vi "AlliGator Get Optimal IRF from Decay v2.vi"(8 "error in (no error)":errorcluster, 11 "Selected Plot Info":T4={"Multiplot XY Graph"=refnum, "Mouse Coordinates"={"Horizontal"=0, "Vertical"=0}, "Plot Index"=-1}) -> (0 "Error Out":errorcluster, 1 "Message Style":T2={"Font"="Consolas", "Text Color"=enum."Black", "Text Background Color"=enum."White", "Text Style"=enum."Regular", "Font Size (Points)"=10.0, "Text Alignment"=0} {"Text Alignment" items=["Left", "Right", "Center"]}, 2 "Message":string, 3 "Extracted IRF":cluster{"t Array":dbl[], "IRF Array":dbl[]})   [LabVIEW 2021, in "AlliGator Decay Analysis.lvlib" / "AlliGator IRF.lvlib"]
doc: "Extract IRF from single-exponential decay by deconvolution and optimization of the time constant."
uses:
  AlliGator IRF.lvlib
  Graphs/XY Graph/XY Graph Selected Plot Info.ctl
  Graphs/XY Graph/XY Graph Refnum.ctl
  <vilib>/Utility/miscctls.llb/LVPoint32TypeDef.ctl
  Rich Text Box/Text Formatting.ctl
  Rich Text Box/Text Colors.ctl
  AlliGator Settings List.ctl
  AlliGator IRF Optimization Controls.ctl
  AlliGator IRF Deconvolution Metrics.ctl
  Fits/IRF(X)PSED/IRF(X)PSED Fixed Parameters v3.ctl
  Fits/IRF(X)PSED/IRF(X)PSED Extraction Options.ctl
  Fits/IRF(X)PSED/Fourier Series Smoothing Option.ctl
  Fits/IRF(X)PSED/Fourier Series Truncation.ctl
  Fits/IRF(X)PSED/IRF Extraction Method.ctl
  Variant/Variant to Data/Variant to I32.vi
  Graphs/XY Graph/XY Graph Add Single Plot with Name.vi
  Graphs/XY Graph/XY Graph Add-Ons.lvlib
  AlliGator Settings.lvlib
  Notebook/Notebook.lvlib
  Fits/Fits.lvlib
  Variant/Variant to Data/Variant to Data.lvlib
  Rich Text Box/Rich Text Box.lvlib
panel:
  in  "Tab Control":T1(tab)
  out "Optimization Graph":cluster{"X Array":dbl[], "Y Array":dbl[]}[](graph)
  out "Power Spectrum Graph":dbl[][](graph)
  in  "Plot Names":string[](array[string])=["Tail Average", "Tail Average SG", "Tail SDV", "Tail SDV S-G", "Tail Max", "Tail Max S-G", "Tail SDV x Average", "Tail SDV x Average S-G", "Slope"]
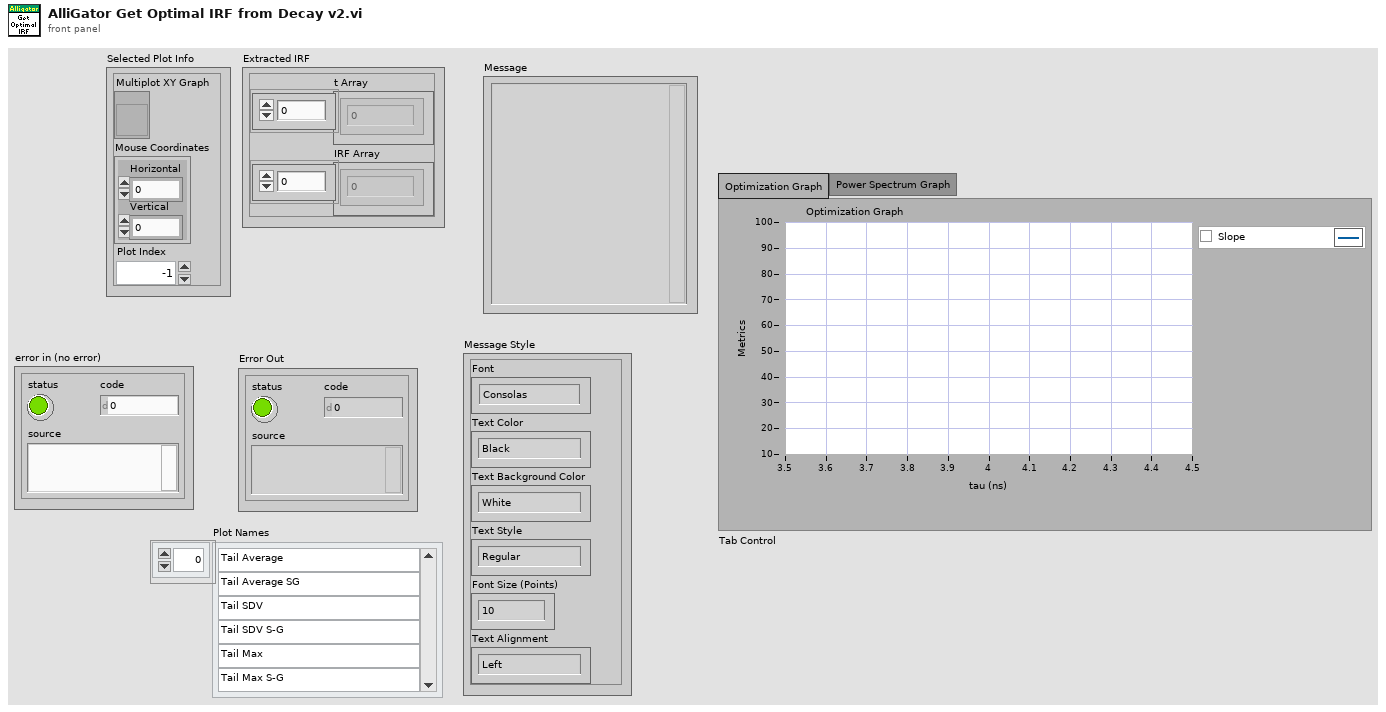
[diagram p1: front panel]
types:
  T1 = enum32{"Optimization Graph", "Power Spectrum Graph"}
  T2 = typedef "Rich Text Box.lvlib/Text Formatting.ctl" = cluster{"Font":string, "Text Color":T3, "Text Background Color":T3, "Text Style":enum16{"Regular", "Bold", "Italic", "Underline", "Strikeout"}, "Font Size (Points)":dbl, "Text Alignment":i32}
  T3 = typedef "Rich Text Box.lvlib/Text Colors.ctl" = enum16{"Unchanged", "Black", "Blue", "Brown", "Gray", "Green", "Orange", "Pink", "Red", "White"}
  T4 = typedef "XY Graph Add-Ons.lvlib/XY Graph Selected Plot Info.ctl" = cluster{"Multiplot XY Graph":T5, "Mouse Coordinates":T6, "Plot Index":i32}
  T5 = typedef "XY Graph Add-Ons.lvlib/XY Graph Refnum.ctl" = refnum<vi>
  T6 = typedef "LVPoint32TypeDef.ctl" = cluster{"Horizontal":i32, "Vertical":i32}
  T7 = typedef "Fits.lvlib/IRF(X)PSED Extraction Options.ctl" = cluster{"Time Constant for IRF Extraction":dbl[unit], "IRF Order":i32, "Fourier Series Smoothing":T8, "Noise Threshold":dbl, "Smoothing Width":dbl, "Fourier Series Truncation":T9, "Truncation Order":i32, "Save Power Spectrum":bool, "Smoothing":bool, "Smoothing Parameter":dbl, "Smoothing Order":u32, "Method":T10}
  T8 = typedef "Fits.lvlib/Fourier Series Smoothing Option.ctl" = enum16{"None", "Lanczos Factors", "Fejer Summation"}
  T9 = typedef "Fits.lvlib/Fourier Series Truncation.ctl" = enum16{"Automatic", "Fixed"}
  T10 = typedef "Fits.lvlib/IRF Extraction Method.ctl" = enum16{"Direct", "Topless", "Toeplitz"}
  T11 = typedef "Fits.lvlib/IRF(X)PSED Fixed Parameters v3.ctl" = cluster{"order":i32, "T":dbl, "Time Constant Array":dbl[], "{S_k, C_k, phi_k, e_k} arrays":cluster{"S_k Array":dbl[], "C_k Array":dbl[], "phi_k Array":dbl[], "e_k Array":dbl[]}, "IRF Extraction Options":T7}
  T12 = typedef "AlliGator Settings.lvlib/AlliGator Settings List.ctl" = enum16{"GUI:Visible Settings Tab", "GUI:Last Run Version", "Source Image:Use Image Histogram for Contrast", "Source Image:Low Count Pixels Rejection Options", "Source Image:High Count Pixels Rejection Options", "Source Image:Use Image Brightness", "Source Image:Blend Overlay with Image Background", "Source Image:Use Fixed ROI Diameter", "Source Image:ROI Diameter", "Source Image:ROI Center Color", "Source Image:Peak Threshold", "Source Image:Intensity Threshold", "Source Image:Image Binning Options", "Source Image:Image Smoothing Options", "Source Image:Image Histogram Active", "Source Image:Invert Binary Mask", "Source Image:Hot Pixel Removal", "Source Image:Overlay Analyzed ROI Center", "Source Image:Auto-Adjust Contrast", "Source Image:Histogram Lower Percentile", "Source Image:Histogram Upper Percentile", "Source Image:Save Source Image", "Source Image:Scale Bar Options", "Source Image:Image Resolution (Pixel Size)", "Source Image:Flatfield Correction", "Data Information:Gate Width", "Data Information:Nanotime Gate Separation", "Data Information:Macrotime Gate Separation", "Data Information:Gate Step", "Data Information:# Gates", "Data Information:Gate Image Exposure", "Data Information:Gate Image Integration", "Data Information:Gates to Skip", "Data Information:Gates to Keep", "Data Information:Define Gates to", "Data Information:Channel Name", "Data Information:Available Channel Names", "Data Information:Channel Arithmetic", "Data Information:Background File Subtraction", "Data Information:Background File", "Data Information:Background Scaling Factor", "Data Information:Background Pile-up Correction", "Data Information:Background Pixel Well Capacity", "Data Information:Laser Period", "Data Information:SYNC Period", "Data Information:Pile-up Correction", "Data Information:Pixel Well Capacity", "Data Information:Dataset Scaling Factor", "Fluorescence Decay_Decay Pre-Processing:Reverse Gates", "Fluorescence Decay_Decay Pre-Processing:Verbose Decay Pre-Processing", "Fluorescence Decay_Decay Pre-Processing:Use Decay Pre-Processing", "Fluorescence Decay_Decay Pre-Processing:Background Subtraction", "Fluorescence Decay_Decay Pre-Processing:Background Definition Range", "Fluorescence Decay_Decay Pre-Processing:Baseline Subtraction Method", "Fluorescence Decay_Decay Pre-Processing:Operations Order", "Fluorescence Decay_Decay Pre-Processing:Smoothing Parameter", "Fluorescence Decay_Decay Pre-Processing:Shift Decay", "Fluorescence Decay_Decay Pre-Processing:Decay Shift Parameters", "Fluorescence Decay_Decay Pre-Processing:Fold Decay", "Fluorescence Decay_Decay Pre-Processing:# Folds", "Fluorescence Decay_Decay Pre-Processing:1-Normalize Decay", "Fluorescence Decay_Decay Pre-Processing:[0-1]-Normalize Decay", "Fluorescence Decay_Decay Pre-Processing:Smoothen Decay", "Fluorescence Decay_Decay Pre-Processing:Extrapolate Decay", "Fluorescence Decay_Decay Pre-Processing:Use Periodicity", "Fluorescence Decay_Decay Pre-Processing:Use Cursors", "Fluorescence Decay_Decay Pre-Processing:Tail Fraction", "Fluorescence Decay_Decay Pre-Processing:Head Fraction", "Fluorescence Decay_Decay Pre-Processing:Additional Points", "Fluorescence Decay_Decay Pre-Processing:Straighten Decay", "Fluorescence Decay_Decay Pre-Processing:Constant Background", "Fluorescence Decay_Decay Pre-Processing:Pixel-Normalize Decay", "Fluorescence Decay_Advanced Analysis:Extract IRF instead of Decay", "Fluorescence Decay_Advanced Analysis:IRF Extraction Options", "Fluorescence Decay_Advanced Analysis:IRF Optimization Options", "Fluorescence Decay_Advanced Analysis:Square Pulse Options", "Fluorescence Decay_Advanced Analysis:IRF Order", "Fluorescence Decay_Advanced Analysis:IRF Time Constants", "Fluorescence Decay_Advanced Analysis:Wavelet Analysis Options", "Fluorescence Decay_Advanced Analysis:Average Lifetime Options", "Fluorescence Decay_Fit Options:Fit Options", "Fluorescence Decay_Fit Options:Use Legacy Fitting Approach", "Fluorescence Decay_Fit Options:Use Data Information Laser Period", "Fluorescence Decay_Fit Parameters:Displayed Fit Parameters", "Fluorescence Decay_Fit Parameters:Fit Parameter Constraints", "Fluorescence Decay_Fit Parameters:Export Tabulated Results", "Fluorescence Decay_Fit Parameters:MLE Baseline Offset Type", "Fluorescence Decay_Fit Parameters:MLE Baseline Offset", "Fluorescence Decay_Fit Parameters:Guess Parameter Names", "Fluorescence Decay_Fit Parameters:Guess Parameter Values", "Fluorescence Decay_Fit Parameters:Guess Parameters Options", "Fluorescence Decay_Styles:Show Last Decay Only", "Fluorescence Decay_Styles:Decay Graph Color Array", "Fluorescence Decay:Decay Graph Active", "Fluorescence Decay Statistics:Min Peak Value", "Fluorescence Decay Statistics:Reject Low Decay Peak Pixels", "Fluorescence Decay Statistics:Reject High Decay Peak Pixels", "Fluorescence Decay Statistics:Max Peak Value", "Time Traces:Use File Timestamp", "Time Traces:Time Step", "Time Traces:Use Intensity Correction File", "Time Traces:Intensity Correction File", "Phasor Plot:Phasor Plot Smoothing Options", "Phasor Plot:Phasor Plot Size", "Phasor Plot:Phasor Plot Graphics Options", "Phasor Plot:Cumulative Phasor Plot", "Phasor Plot:Use Phasor Brightness", "Phasor Plot:Blend Overlay with Phasor Background", "Phasor Plot:Save Phasor Plot", "Phasor Plot:Show References", "Phasor Plot:Phasor Ratio Decay Range", "Phasor Plot:Exponential Fading", "Phasor Plot:Phasor Ratio Reference Colors", "Phasor Plot:Reference Radius", "Phasor Plot:Show Color Map Vertices", "Phasor Plot:Phasor Plot Active", "Phasor Plot:Phasor Ratio Color Map Type", "Phasor Plot:Phasor Ratio Color Map", "Phasor Plot:Phasor Ratio Display Range", "Phasor Plot:Selected Image ROI(s)", "Phasor Plot:All Image ROIs", "Phasor Plot:Selected Phasor Plot ROI(s)", "Phasor Plot:All Phasor Plot ROIs", "Phasor Plot:Phasor Ratio Color-Coded Quantity", "Phasor Plot:Store Phasor Harmonics", "Phasor Plot:Draw Reference Segment", "Phasor Plot:User-Defined Quantity", "Phasor Graph:Phasor Frequency", "Phasor Graph:Phasor Ratio Type", "Phasor Graph:Pixel-level Phasor Computation", "Phasor Graph:Save Phasor Graph", "Phasor Graph:Phasor Graph Active", "Phasor Graph:Phasor SDV Options", "Phasor Calibration:Use Backup Calibration if needed", "Phasor Graph:Define Shortest Lifetime as", "Phasor Calibration:Backup Calibration Type", "Phasor Calibration:Calibration Type", "Phasor Calibration:Calibration Lifetime", "Phasor Calibration:Calibration Map Algorithm", "Single-Exponential Phasor Locus (SEPL):Gate Parameters", "Single-Exponential Phasor Locus (SEPL):User-defined Gate", "Single-Exponential Phasor Locus (SEPL):User-defined IRF", "Single-Exponential Phasor Locus (SEPL):Phasor Parameters", "Single-Exponential Phasor Locus (SEPL):Decay & IRF Parameters", "Single-Exponential Phasor Locus (SEPL):Display Parameters", "Lifetime Analysis:Decay Analysis Parameters", "Lifetime Analysis:Lifetime Map Active", "Plugins:Python Settings", "Miscellaneous:Verbose Mode", "Miscellaneous:Beep after Script", "Miscellaneous:Saved Image File Format", "Miscellaneous:Exported Gate Image Settings", "Miscellaneous:Include Loading in Timing", "Miscellaneous:Verbose Settings Mode", "Miscellaneous:Histogram Options", "Miscellaneous:Beep on Error", "Miscellaneous:# Logical Processors Used", "Miscellaneous:ROI Description Max Characters", "Miscellaneous:Verbose Error Mode", "Miscellaneous:Transparent Mask Color"}
  T13 = typedef "AlliGator Decay Analysis.lvlib/AlliGator IRF.lvlib/AlliGator IRF Optimization Controls.ctl" = cluster{"Search Range":dbl[unit], "Search Step":dbl[unit], "Tail threshold (%)":dbl, "Regularized IRF":bool, "Export Plot":bool, "Export Data":bool, "Smooth Metrics":bool, "S-G Side Points":i32, "S-G Polynomial Order":i32, "Metrics":T14}
  T14 = typedef "AlliGator Decay Analysis.lvlib/AlliGator IRF.lvlib/AlliGator IRF Deconvolution Metrics.ctl" = enum16{"Average", "SDV", "Max", "Average * SDV", "Slope"}
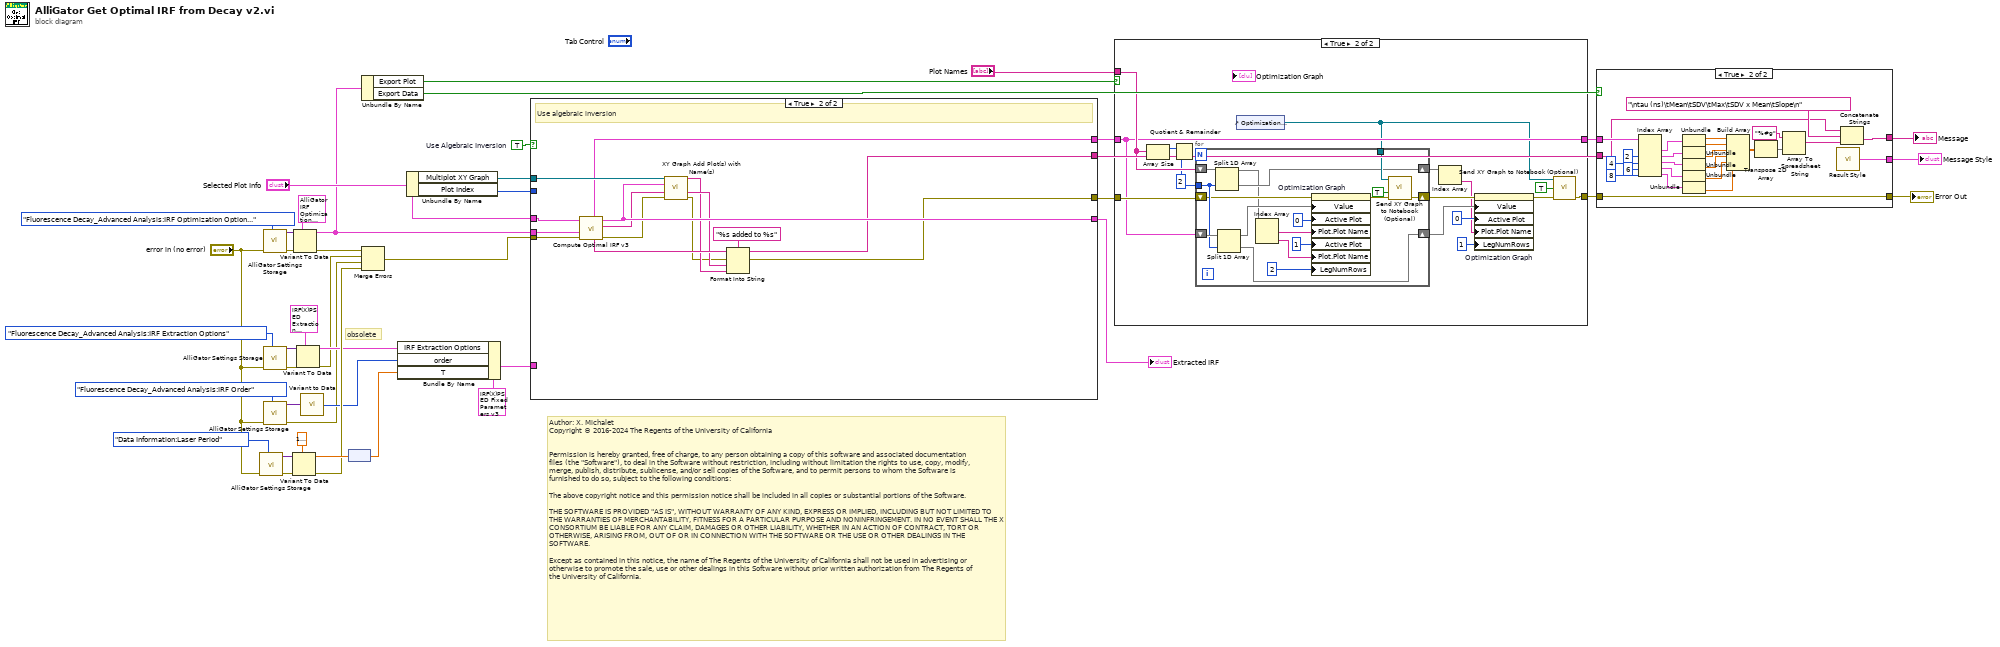
[diagram p0: block diagram]
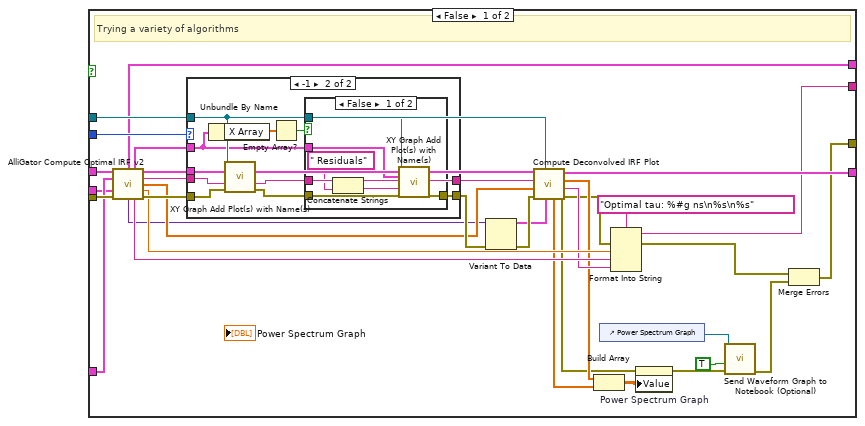
[diagram p4: hidden frame]
diagram:
  w13 = TRUE  # Use Algebraic Inversion
  # "Author: X. Michalet\nCopyright © 2016-2024 The Regents of the University of California\n \n\nPermission is hereby granted, free of charge, to any person obtaining a copy of this software and associated documentation files (the \"Software\"), to deal in the Software without restriction, including without limitation the rights to use, copy, modify, merge, publish, distribute, sublicense, and/or sell copies of the Software, and to permit persons to whom the Software is furnished to do so, subject to the following conditions:\n\nThe above copyright notice and this permission notice shall be included in all copies or substantial portions of the Software.\n\nTHE SOFTWARE IS PROVIDED \"AS IS\", WITHOUT WARRANTY OF ANY KIND, EXPRESS OR IMPLIED, INCLUDING BUT NOT LIMITED TO THE WARRANTIES OF MERCHANTABILITY, FITNESS FOR A PARTICULAR PURPOSE AND NONINFRINGEMENT. IN NO EVENT SHALL THE X CONSORTIUM BE LIABLE FOR ANY CLAIM, DAMAGES OR OTHER LIABILITY, WHETHER IN AN ACTION OF CONTRACT, TORT OR OTHERWISE, ARISING FROM, OUT OF OR IN CONNECTION WITH THE SOFTWARE OR THE USE OR OTHER DEALINGS IN THE SOFTWARE.\n\nExcept as contained in this notice, the name of The Regents of the University of California shall not be used in advertising or otherwise to promote the sale, use or other dealings in this Software without prior written authorization from The Regents of the University of California."
  # "obsolete"
  n1 = call "AlliGator Settings Storage.vi"("AlliGator Settings List"=AlliGator_Settings_List."Data Information:Laser Period", "Error In"="error in (no error)") -> ("Error Out"=w33:errorcluster, "Variant Data out"=w35:variant)  [unwired: 8 in]
  n2 = call "AlliGator Settings Storage.vi"("AlliGator Settings List"=AlliGator_Settings_List."Fluorescence Decay_Advanced Analysis:IRF Optimization Options", "Error In"="error in (no error)") -> ("Error Out"=w41:errorcluster, "Variant Data out"=w42:variant)  [unwired: 8 in]
  n3 = call "AlliGator Settings Storage.vi"("AlliGator Settings List"=AlliGator_Settings_List."Fluorescence Decay_Advanced Analysis:IRF Extraction Options", "Error In"="error in (no error)") -> ("Error Out"=w27:errorcluster, "Variant Data out"=w28:variant)  [unwired: 8 in]
  n4 = call "AlliGator Settings Storage.vi"("AlliGator Settings List"=AlliGator_Settings_List."Fluorescence Decay_Advanced Analysis:IRF Order", "Error In"="error in (no error)") -> ("Error Out"=w20:errorcluster, "Variant Data out"=w26:variant)  [unwired: 8 in]
  n5 = Variant To Data(error in=w33, type=dbl[unit] 1e-09 ("Time Constant"), Variant=w35) -> (data=w32:dbl[unit], error out=w30:errorcluster)
  n6 = Variant To Data(error in=w41, type=T13 {"Search Range"=1e-09, "Search Step"=1e-09, "Tail threshold (%)"=1.0, "Regularized IRF"=FALSE, "Export Plot"=FALSE, "Export Data"=FALSE, "Smooth Metrics"=FALSE, "S-G Side Points"=1, "S-G Polynomial Order"=3, "Metrics"=enum."Average"} ("IRF Optimization Control"), Variant=w42) -> (data=w12:T13, error out=w38:errorcluster)
  n7 = Variant To Data(error in=w27, type=T7 {"Time Constant for IRF Extraction"=4.08e-09, "IRF Order"=132, "Fourier Series Smoothing"=enum."Fejer Summation", "Noise Threshold"=0.1, "Smoothing Width"=0.1, "Fourier Series Truncation"=enum."Automatic", "Truncation Order"=0, "Save Power Spectrum"=FALSE, "Smoothing"=FALSE, "Smoothing Parameter"=0.0, "Smoothing Order"=1, "Method"=enum."Direct"} ("IRF Extraction Options"), Variant=w28) -> (data=w23:T7, error out=w21:errorcluster)
  n8 = call-poly "Variant to Data.vi"("Variant"=w26) -> ("Value"=w22:i32)  [unwired: 8 in]
  n9 = node(w32) -> (w19:dbl)
  n10 = Unbundle By Name(w12) -> ("Export Plot"=w9:bool, "Export Data"=w8:bool)
  n11 = Merge Errors(w38, w21, w20, w30) -> (w31:errorcluster)
  n12 = Bundle By Name(cluster=T11 {"order"=0, "T"=0.0, "Time Constant Array"=[], "{S_k, C_k, phi_k, e_k} arrays"={"S_k Array"=[], "C_k Array"=[], "phi_k Array"=[], "e_k Array"=[]}, "IRF Extraction Options"={"Time Constant for IRF Extraction"=1e-18, "IRF Order"=0, "Fourier Series Smoothing"=enum."None", "Noise Threshold"=0.0, "Smoothing Width"=0.0, "Fourier Series Truncation"=enum."Automatic", "Truncation Order"=0, "Save Power Spectrum"=FALSE, "Smoothing"=FALSE, "Smoothing Parameter"=0.0, "Smoothing Order"=1, "Method"=enum."Direct"}} ("IRF*PSED Fixed Parameters"), "IRF Extraction Options"=w23, "order"=w22, "T"=w19) -> (w15:T11)
  n13 = Unbundle By Name("Selected Plot Info") -> ("Multiplot XY Graph"=w16:T5, "Plot Index"=w17:i32)
  n14 = case shown="True" w13 {
    tunnel: "Selected Plot Info" -> [w75 w110]
    tunnel: [w74 w108] -> w37
    tunnel: w31 -> [w73 w111]
    tunnel: w17 -> [w72 _]
    tunnel: w16 -> [w71 w109]
    tunnel: [w66 w100] -> w10
    tunnel: w15 -> [w62 _]
    tunnel: w12 -> [w46 w99]
    tunnel: [w45 w98] -> w11
    tunnel: [w44 w97] -> w4
    frame False {
      # "Trying a variety of algorithms"
      n15 = call "AlliGator Compute Optimal IRF v2.vi"("Selected Plot Info"=w75, "IRF*PSED Fixed Parameters"=w62, "IRF Optimization Control"=w46, "Error In"=w73) -> ("Optimization Graph"=w45:cluster{"Ramp Pattern":dbl[], dbl[]}[], "Residuals Plot"=w65:cluster{"X Array":dbl[], "Y Array":dbl[]}, "Fitted Plot"=w70:cluster{"X Array":dbl[], "Y Array":dbl[]}, "Plot Name"=w69:string, "Fit Parameter Values"=w57:dbl[], "Optimal Tau"=w63:dbl, "Additional Data"=w56:variant, "Fit Results String"=w64:string, "Error Out"=w68:errorcluster)  [unwired: 3 in]
      n16 = case shown="-1" w72 {
        tunnel: w71 -> [_ w81]
        tunnel: w70 -> [_ w88]
        tunnel: w69 -> [w78 w87]
        tunnel: w68 -> [w77 w86]
        tunnel: [w78 w79] -> w67
        tunnel: [w77 w82] -> w61
        tunnel: w65 -> [_ w80]
        frame 0, Default {
          # "if programmatic do not plot the fit\nbut the IRF  only"
        }
        frame -1 {
          n17 = Unbundle By Name(w80) -> ("X Array"=w85:dbl[])
          n18 = call-poly "XY Graph Add Plot(s) with Name(s).vi"("XYGraph Ref in"=w81, "Plot"=w88, "Plot Name (\"Plot\")"=w87, "error in (no error)"=w86) -> ("Plot Name"=w79:string, "error out"=w83:errorcluster)  [unwired: 8 in, 2 out]
          n19 = Empty Array?(array=w85) -> (empty?=w84:bool)
          n20 = case shown="False" w84 {
            tunnel: w83 -> [w95 w96]
            tunnel: [w94 w96] -> w82
            tunnel: w81 -> [w93 _]
            tunnel: w80 -> [w92 _]
            tunnel: w79 -> [w91 _]
            frame False {
              n21 = Concatenate Strings(w91, " Residuals" ("string")) -> (w89:string)
              n22 = call-poly "XY Graph Add Plot(s) with Name(s).vi"("XYGraph Ref in"=w93, "Plot"=w92, "Plot Name (\"Plot\")"=w89, "error in (no error)"=w95) -> ("error out"=w94:errorcluster)  [unwired: 8 in, 3 out]
            }
            frame True {
            }
          }
        }
      }
      n23 = Variant To Data(error in=w61, Variant=w56) -> (data=w59:T11, error out=w60:errorcluster)  [unwired: 1 in]
      n24 = call "Compute Deconvolved IRF Plot.vi"("IRF*PSED fixed Parameters"=w59, "XYGraph in"=w71, "error in (no error)"=w60, "Fit Parameter Values"=w57, "Plot Name"=w67, "Fitted Decay"=w70) -> ("error out"=w54:errorcluster, "Amplitude String"=w58:string, "Power Spectrum"=w55:dbl[], "IRF Plot"=w74:cluster{"X Array":dbl[], "Y Array":dbl[]}, "Smoothed Power Spectrum"=w49:dbl[])  [unwired: 1 in]
      n25 = Build Array(w55, w49) -> (w47:dbl[][])
      n26 = control-ref of="Power Spectrum Graph"() -> (w51:refnum<vi>)
      n27 = Format Into String(format string="Optimal tau: %#g ns\n%s\n%s", error in=w54, w63, w64, w58) -> (resulting string=w44:string, error out=w48:errorcluster)  [unwired: 1 in]
      n28 = property on="Power Spectrum Graph" class="WFGraph (strict)"(error in=w54, "Value"=w47) -> (error out=w53:errorcluster)  [unwired: 1 in, 1 out]
      n29 = call "Send Waveform Graph to Notebook (Optional).vi"("error in (no error)"=w53, "Send Graph to Notebook?"=TRUE, "Multiwaveform Graph Refnum"=w51) -> ("error out"=w50:errorcluster)  [unwired: 8 in]
      n30 = Merge Errors(w48, w50) -> (w66:errorcluster)
    }
    frame True {
      # "Use algebraic inversion"
      n31 = call "Compute Optimal IRF v3.vi"("Error In"=w111, "IRF Optimization Control"=w99, "Selected Plot Info"=w110) -> ("Error Out"=w106:errorcluster, "Plot Name"=w107:string, "IRF Plot"=w108:cluster{"X Array":dbl[], "Y Array":dbl[]}, "Optimal IRF Results String"=w105:string, "Optimization Graph"=w98:cluster{dbl[], dbl[]}[])  [unwired: 3 in, 1 out]
      n32 = call-poly "XY Graph Add Plot(s) with Name(s).vi"("XYGraph Ref in"=w109, "Plot"=w108, "Plot Name (\"Plot\")"=w107, "error in (no error)"=w106) -> ("XY Graph Caption (or Label)"=w102:string, "Plot Name"=w104:string, "error out"=w101:errorcluster)  [unwired: 8 in, 1 out]
      n33 = Format Into String(format string="%s added to %s", initial string=w105, error in=w101, w104, w102) -> (resulting string=w97:string, error out=w100:errorcluster)
    }
  }
  "Extracted IRF" <- w37
  n34 = case shown="True" w9 {
    tunnel: w11 -> [w112 w124]
    tunnel: w10 -> [w113 w129]
    tunnel: [w113 w123] -> w7
    tunnel: [w112 w124] -> w5
    tunnel: "Plot Names" -> [_ w126]
    frame False {
    }
    frame True {
      w125 = 2 ("y")
      n35 = Array Size(array=w126) -> (size(s)=w128:i32)
      n36 = Quotient & Remainder(x=w128, y=w125) -> (floor(x/y)=w127:i32)  [unwired: 1 out]
      n37 = control-ref of="Optimization Graph"() -> (w122:refnum<vi>)
      n38 = for {
        N: w127 -> [_]
        tunnel: w122 -> [w145]
        shift-right: [w144] -> w121
        shift-left: w129 -> [w139]
        shift-right: [w142] -> w117
        shift-left: w126 -> [w143]
        tunnel: w125 -> [w140]
        shift-right: [w135] -> w119
        shift-left: w124 -> [w141]
        n39 = Split 1D Array(array=w143, index=w140) -> (first subarray=w133:string[], second subarray=w142:string[])
        n40 = Split 1D Array(array=w141, index=w140) -> (first subarray=w137:cluster{"Ramp Pattern":dbl[], dbl[]}[], second subarray=w135:cluster{"Ramp Pattern":dbl[], dbl[]}[])
        n41 = Index Array(array=w133) -> (element #1=w132:string, element #2=w131:string)  [unwired: 2 in]
        n42 = property on="Optimization Graph" class="XYGraph (strict)"(error in=w139, "Value"=w137, "Active Plot"=u32 0, "Plot.Plot Name"=w132, "Active Plot"=u32 1, "Plot.Plot Name"=w131, "LegNumRows"=u32 2 ("Legend:Number of Rows")) -> (error out=w138:errorcluster)  [unwired: 1 in, 1 out]
        n43 = call "Send XY Graph to Notebook (Optional).vi"("error in (no error)"=w138, "Send Graph to Notebook?"=TRUE, "XYGraph in"=w145) -> ("error out"=w144:errorcluster)  [unwired: 8 in]
      }
      n44 = Index Array(array=w117) -> (element=w116:string)  [unwired: 1 in]
      n45 = property on="Optimization Graph" class="XYGraph (strict)"(error in=w121, "Value"=w119, "Active Plot"=u32 0, "Plot.Plot Name"=w116, "LegNumRows"=u32 1 ("Legend:Number of Rows")) -> (error out=w120:errorcluster)  [unwired: 1 in, 1 out]
      n46 = call "Send XY Graph to Notebook (Optional).vi"("error in (no error)"=w120, "Send Graph to Notebook?"=TRUE, "XYGraph in"=w122) -> ("error out"=w123:errorcluster)  [unwired: 8 in]
    }
  }
  n47 = case shown="True" w8 {
    tunnel: w7 -> [w148 w166]
    tunnel: [w148 w166] -> w6
    tunnel: w5 -> [_ w173]
    tunnel: w4 -> [w147 w155]
    tunnel: [w147 w157] -> w3
    tunnel: [_ w156] -> w2
    frame False {
    }
    frame True {
      n48 = Index Array(array=w173, index #2=2 ("index"), index #3=4 ("index"), index #4=6 ("index"), index #5=8 ("index")) -> (element #1=w172:cluster{"Ramp Pattern":dbl[], dbl[]}, element #2=w164:cluster{"Ramp Pattern":dbl[], dbl[]}, element #3=w163:cluster{"Ramp Pattern":dbl[], dbl[]}, element #4=w159:cluster{"Ramp Pattern":dbl[], dbl[]}, element #5=w151:cluster{"Ramp Pattern":dbl[], dbl[]})  [unwired: 1 in]
      n49 = Unbundle(w172) -> ("Ramp Pattern"=w171:dbl[], w170:dbl[])
      n50 = Unbundle(w164) -> (w162:dbl[])  [unwired: 1 out]
      n51 = Unbundle(w163) -> (w161:dbl[])  [unwired: 1 out]
      n52 = Unbundle(w159) -> (w158:dbl[])  [unwired: 1 out]
      n53 = Unbundle(w151) -> (w149:dbl[])  [unwired: 1 out]
      n54 = Build Array(w171, w170, w162, w161, w158, w149) -> (w169:dbl[][])
      n55 = Transpose 2D Array(2D array=w169) -> (transposed array=w165:dbl[][])
      n56 = Array To Spreadsheet String(array=w165, 3:"%#g" ("format string")) -> (spreadsheet string=w167:string)  [unwired: 1 in]
      n57 = call "Result Style.vi"() -> ("Default Text Formatting"=w156:T2)
      n58 = Concatenate Strings(w155, "\ntau (ns)\tMean\tSDV\tMax\tSDV x Mean\tSlope\n" ("string"), w167) -> (w157:string)
    }
  }
  "Error Out" <- w6
  "Message" <- w3
  "Message Style" <- w2
